vi "send_command.vi"(8 "error in (no error)":errorcluster, 10 "command":string, 11 "VISA Refnum in":refnum<visa-resource-name>) -> (0 "error out":errorcluster, 1 "Return Byte Array":u8[](array[numeric]), 2 "return string":string, 3 "VISA resource name out":refnum<visa-resource-name>)   [LabVIEW 2018]
doc: "send the command to the serial port and return the answer as string and as byte array"
uses:
  12c73bc9-6aab-4fb1-a36f-f980820021b3.vi
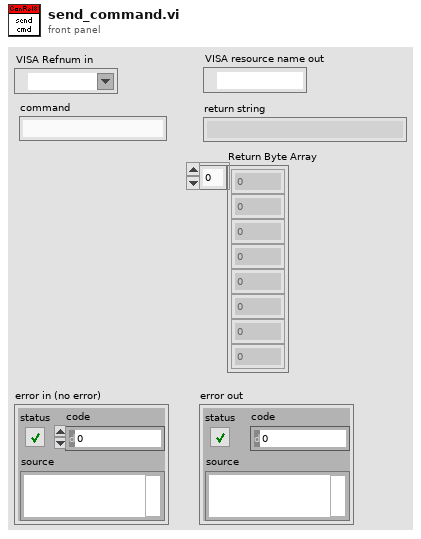
[diagram p1: front panel]
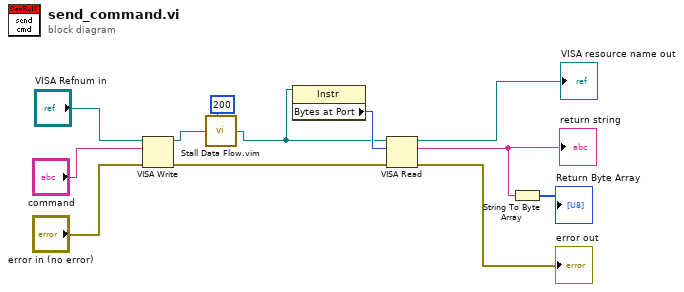
[diagram p0: block diagram]
diagram:
  n1 = VISA Write(VISA resource name="VISA Refnum in", write buffer="command", error in (no error)="error in (no error)") -> (VISA resource name out=w5:refnum<visa-resource-name>, error out=w3:errorcluster)  [unwired: 1 out]
  n2 = call "Stall Data Flow.vim"("value in"=w5, "milliseconds to wait"=u32 200) -> ("value out"=w9:refnum<visa-resource-name>)  [unwired: 1 out]
  n3 = property class="Instr"(reference=w9) -> ("Bytes at Port"=w10:u32)  [unwired: 1 in, 2 out]
  n4 = VISA Read(VISA resource name=w9, byte count=w10, error in (no error)=w3) -> (VISA resource name out=→"VISA resource name out":refnum<visa-resource-name>, read buffer=w8:string, error out=→"error out":errorcluster)  [unwired: 1 out]
  "return string" <- w8
  n5 = String To Byte Array(string=w8) -> (unsigned byte array=→"Return Byte Array":u8[])
